vi "FTW-Example-Actors-RT.vi"() -> ()   [LabVIEW 2013]
uses:
  source/actor/Connector/FTW-ActorConnector.lvclass
  source/actor/Ether/FTW-Ether.lvclass
panel:
  in  "Boolean":bool
  out "Instance Inbox Address":string
  out "Initialized Response":string
  out "Timed out?":bool
  out "Ping Response":string
  in  "FTW Ether Configuration":string="{\n  \"ApplicationName\": \"Actor Example\",\n  \"ApplicationVersion\": \"0.1.0-1\",\n  \"LoggerAddress\": \"inproc://*\",\n  \"LoggerName\": \"ActorExample\",\n  \"LoggerDirectory\": \"/c/logs\",\n  \"LoggerDiskThrashDelay\": 200\n}"
  in  "Actor 1 Configuration":string="{\n  \"Identity\": \"FeatherweightActorExample\",\n  \"InboxAddress\": \"inproc://*\",\n  \"LoggerAddress\": \"\",\n  \"DebugEnableInboxLogging\": false,\n  \"DebugEnableJobLogging\": false,\n  \"DebugShowPanel\": false\n}"
  out "error out":errorcluster
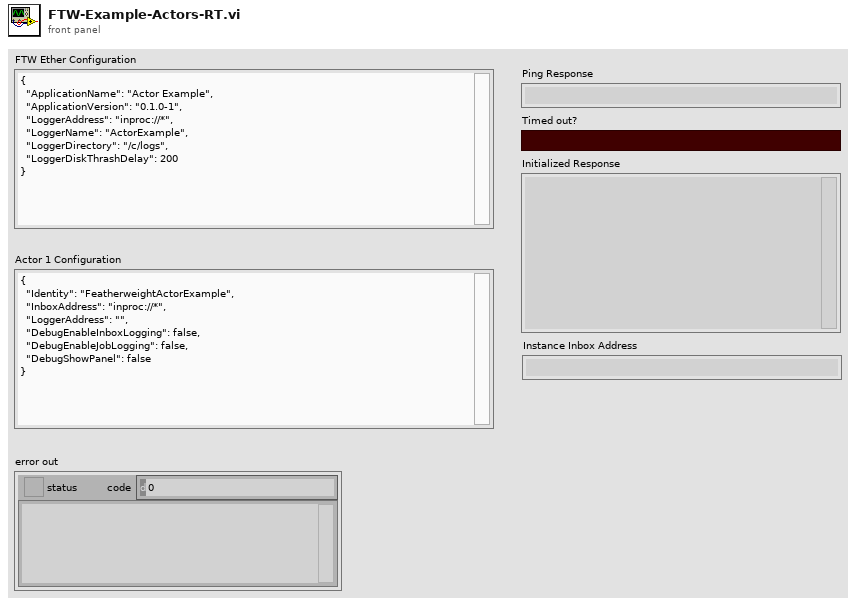
[diagram p1: front panel]
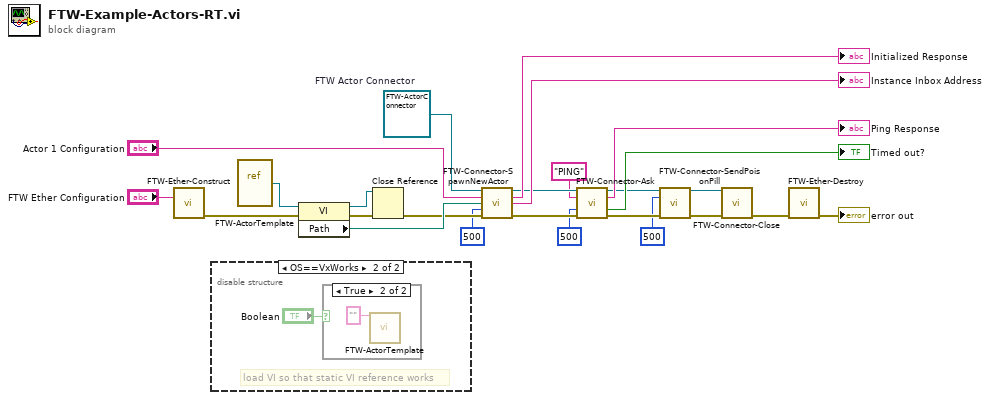
[diagram p0: block diagram]
diagram:
  w16 = refnum<class "FTW-ActorConnector.lvclass"> refnum  # FTW Actor Connector
  n1 = call "FTW-Ether-Construct.vi"("FTW Ether Configuration"="FTW Ether Configuration") -> ("error out"=w24:errorcluster)  [unwired: 14 in]
  n2 = disable-structure shown="OS==VxWorks" {
    frame condition #0 (active) {
    }
    frame condition #1 {
      # "load VI so that static VI reference works"
      n3 = case shown="True" "Boolean" {
        frame False {
        }
        frame True {
          n4 = call "FTW-ActorTemplate.vi"("FTW Actor Instance Configuration"="") -> ()  [unwired: 14 in, 1 out]
        }
      }
    }
  }
  n5 = vi-ref "FTW-ActorTemplate.vi"() -> (w15:refnum<vi>)
  n6 = property class="VI"(reference=w15, error in=w24) -> (reference out=w5:refnum<vi>, error out=w4:errorcluster, "Path"=w14:path)
  n7 = Close Reference(reference=w5, error in (no error)=w4) -> (error out=w3:errorcluster)
  n8 = call "FTW-Connector-SpawnNewActor.vi"("FTW Actor Connector Type"=w16, "Configuration"="Actor 1 Configuration", "Actor VI Filepath"=w14, "Timeout"=500, "error in"=w3) -> ("FTW Actor Connector"=w13:refnum<class "FTW-ActorConnector.lvclass">, "Initialized Response"=→"Initialized Response":string, "Instance Inbox Address"=→"Instance Inbox Address":string, "error out"=w12:errorcluster)  [unwired: 7 in]
  n9 = call "FTW-Connector-Ask.vi"("FTW Actor Connector"=w13, "Request Header"="PING", "Timeout"=500, "error in"=w12) -> ("FTW Actor Connector out"=w10:refnum<class "FTW-ActorConnector.lvclass">, "Response Header"=→"Ping Response":string, "Timed out?"=→"Timed out?":bool, "error out"=w9:errorcluster)  [unwired: 6 in, 2 out]
  n10 = call-dynamic "FTW-Connector-SendPoisonPill.vi"("FTW Actor Connector"=w10, "Timeout"=500, "error in"=w9) -> ("FTW Actor Connector out"=w8:refnum<class "FTW-ActorConnector.lvclass">, "error out"=w7:errorcluster)  [unwired: 8 in, 3 out]
  n11 = call-dynamic "FTW-Connector-Close.vi"("FTW Actor Connector"=w8, "error in"=w7) -> ("error out"=w20:errorcluster)  [unwired: 13 in]
  n12 = call "FTW-Ether-Destroy.vi"("error in"=w20) -> ("error out"=→"error out":errorcluster)  [unwired: 14 in]
